vi "Reduce Timeout.vi"(8 "error in (no error)":errorcluster, 10 "New Timeout time(ms)":i32, 11 "Interruptible Reply Core in":refnum<class "Interruptible Reply Core.lvclass">) -> (0 "error out":errorcluster, 1 "Timeout time reduced?":bool, 3 "Interruptible Reply Core out":refnum<class "Interruptible Reply Core.lvclass">)   [LabVIEW 2020, in "Publisher.lvlib" / "Interruptible Reply Core.lvclass"]
doc: "Reduce the timeout time on the Response Core if possible."
uses:
  Interruptible Reply Core.lvclass
  Interruptible Reply Core.lvclass/Interruptible Reply Core.ctl
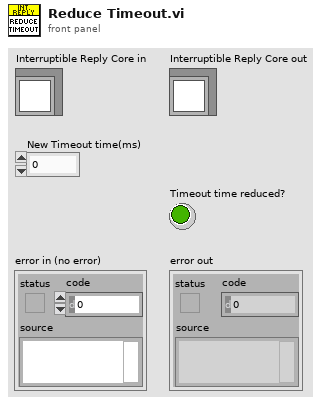
[diagram p1: front panel]
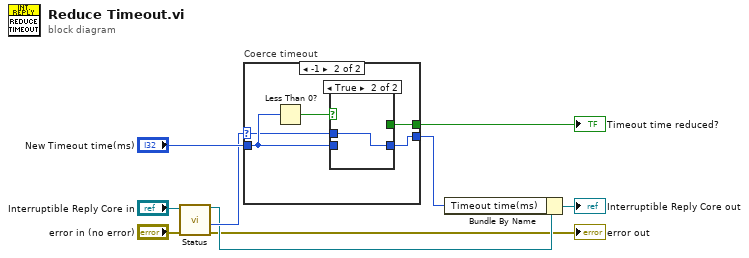
[diagram p0: block diagram]
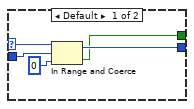
[diagram p2: hidden frame]
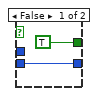
[diagram p3: hidden frame]
diagram:
  n1 = call-dynamic "Status.vi"("error in (no error)"="error in (no error)", "Response Core in"="Interruptible Reply Core in") -> ("error out"=→"error out":errorcluster, "Time to Timeout (ms)"=w7:i32, "Response Core out"=w5:refnum<class "Interruptible Reply Core.lvclass">)  [unwired: 6 in, 1 out]
  n2 = case "Coerce timeout" shown="-1" w7 {
    selector: w7 -> [w12 w15]
    tunnel: [w11 w17] -> w6
    tunnel: "New Timeout time(ms)" -> [w14 w16]
    tunnel: [w10 w18] -> w1
    frame Default {
      n3 = In Range and Coerce(upper limit=w12, x=w14, lower limit=0) -> (coerced(x)=w11:i32, In Range?=w10:bool)
    }
    frame -1 {
      n4 = Less Than 0?(x=w16) -> (x < 0?=w19:bool)
      n5 = case shown="True" w19 {
        tunnel: [TRUE _] -> w18
        tunnel: [w20 w22] -> w17
        tunnel: w16 -> [w20 _]
        tunnel: w15 -> [_ w22]
        frame False {
        }
        frame True {
        }
      }
    }
  }
  "Timeout time reduced?" <- w1
  n6 = Bundle By Name(cluster=w5, "Timeout time(ms)"=w6) -> (→"Interruptible Reply Core out":refnum<class "Interruptible Reply Core.lvclass">)
